vi "New Medlem.vi"(11 "Error in":errorcluster caption="Error in (no error)") -> (4 "New Medlem":refnum<class "Medlem.lvclass">, 15 "Error out":errorcluster)   [LabVIEW 2018, in "HOG Medlem.lvlib" / "Medlem.lvclass"]
doc: "Creates a <B>New Medlem</B> for start with Launch Actor.vi.\n\nThis VI runs only if there is no error on <B>Error in</B>.\n\nSteen Schmidt\nGPower\n12/4 2017"
uses:
  Medlem.lvclass
panel:
  # "#ControlsNeeded (Actor Input Parameters) This VI is optional.\n\nIf this Actor has private data that needs setting when you create a new Actor,\nyou can use this \"New Actor\" VI to set those parameters and get your Actor out\nof. Then use this VI instead of the Actor class constant to create your Actor with."
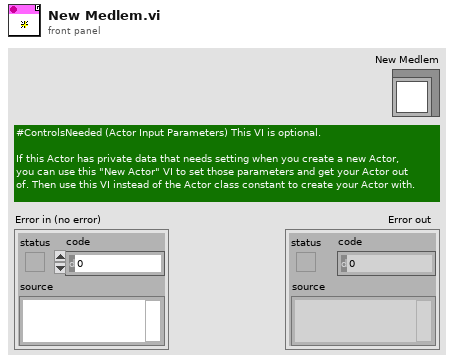
[diagram p1: front panel]
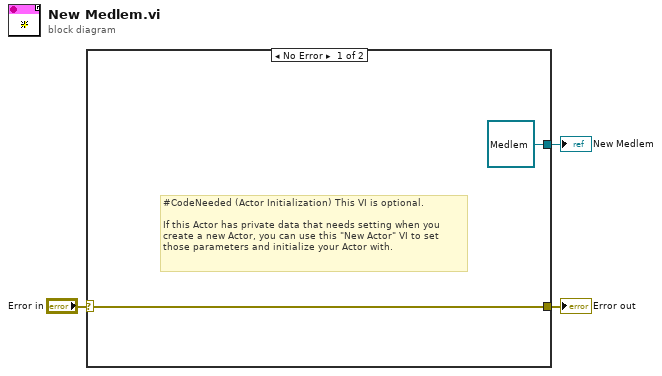
[diagram p0: block diagram]
diagram:
  n1 = case shown="No Error" "Error in" {
    selector: "Error in" -> [w5 w6]
    tunnel: [w5 w6] -> w2
    tunnel: [refnum<class "Medlem.lvclass"> refnum ("New Actor.lvclass") _] -> w1
    frame No Error {
      # "#CodeNeeded (Actor Initialization) This VI is optional.\n\nIf this Actor has private data that needs setting when you\ncreate a new Actor, you can use this \"New Actor\" VI to set\nthose parameters and initialize your Actor with."
    }
    frame Error {
    }
  }
  "New Medlem" <- w1
  "Error out" <- w2
